vi "p8.vi"() -> ()   [LabVIEW 2015]
panel:
  out "floor(x/y)":i32
  out "x-y*floor(x/y)":i32
  out "element":i32
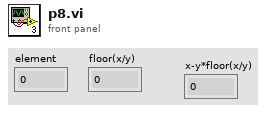
[diagram p1: front panel]
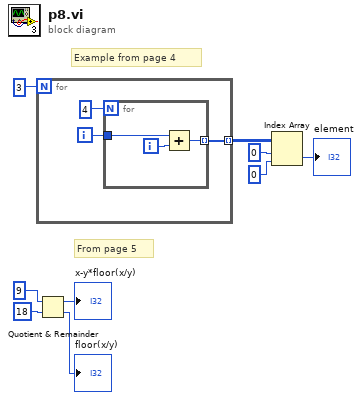
[diagram p0: block diagram]
diagram:
  # "From page 5"
  # "Example from page 4"
  n1 = for {
    N: 3 -> [_]
    tunnel: [w10] -> w7 mode=indexing
    i -> [w11]
    n2 = for {
      N: 4 -> [_]
      tunnel: w11 -> [w14]
      tunnel: [w13] -> w10 mode=indexing
      i -> [w15]
      n3 = Add(x=w14, y=w15) -> (x+y=w13:i32)
    }
  }
  n4 = Quotient & Remainder(x=9, y=18) -> (x-y*floor(x/y)=→"x-y*floor(x/y)":i32, floor(x/y)=→"floor(x/y)":i32)
  n5 = Index Array(array=w7, index (row)=0, index (col)=0) -> (element=→"element":i32)
